vi "GetText.vi"(8 "error in":errorcluster, 11 "Tagbus PID Module editor node in":refnum<class "PID Module editor node.lvclass">) -> (0 "error out":errorcluster, 1 "additional text":string, 2 "text":string, 3 "Tagbus PID Module editor node out":refnum<class "PID Module editor node.lvclass">, 4 "glyph":string)   [LabVIEW 2014, in "PID Module editor node.lvclass"]
uses:
  PID Module editor node.lvclass
  <vilib>/NI/Tag Bus Data Framework/Configuration Editor/Classes/Module editor node/Read display name.vi
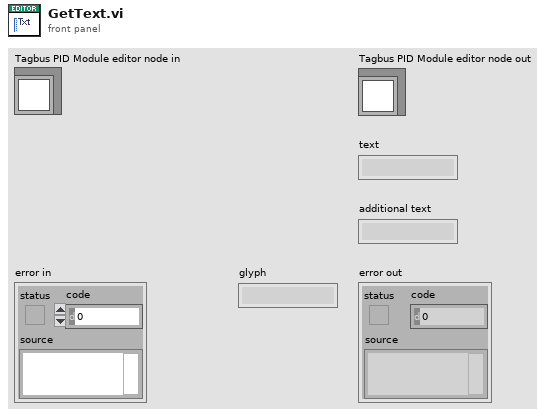
[diagram p1: front panel]
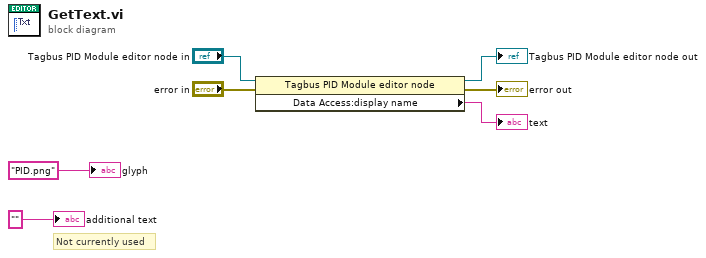
[diagram p0: block diagram]
diagram:
  # "Not currently used"
  n1 = property class="Tagbus PID Module editor node"(reference="Tagbus PID Module editor node in", error in="error in") -> (reference out=→"Tagbus PID Module editor node out":refnum<class "PID Module editor node.lvclass">, error out=→"error out":errorcluster, "Data Access:display name"=→"text":string)
  "additional text" <- "" ("additional text")
  "glyph" <- "PID.png" ("glyph")
